vi "Analog Trigger Detect.vi"(8 "acq.Trigger Invert":bool, 9 "acq.Trigger High":i16, 10 "acq.Trigger Low":i16, 11 "Input Data":i16) -> (2 "Analog Trigger Detect":bool, 3 "Analog Arm Trig":bool)   [LabVIEW 2012]
uses:
  <instrlib>/FlexRIO/Libraries/Helper VIs/NI FlexRIO Helper VIs.lvlib
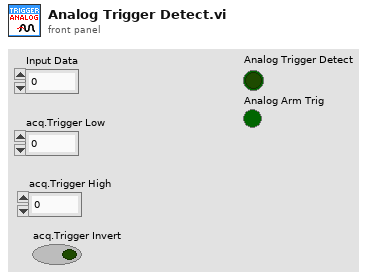
[diagram p1: front panel]
types:
  T1 = cluster{"acq.Trigger Low":i16, "acq.Trigger Invert":bool, "acq.Trigger High":i16}
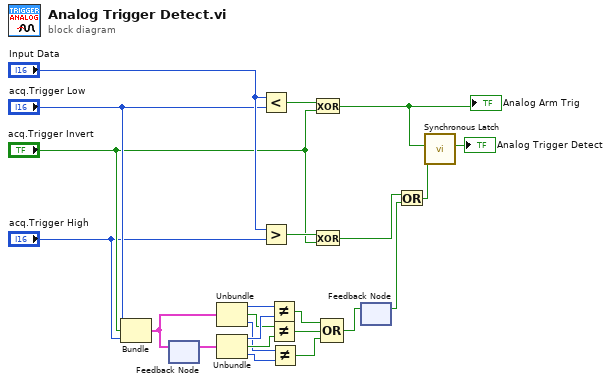
[diagram p0: block diagram]
diagram:
  n1 = Bundle("acq.Trigger Low"="acq.Trigger Low", "acq.Trigger Invert"="acq.Trigger Invert", "acq.Trigger High"="acq.Trigger High") -> (w5:T1)  [unwired: 1 in]
  n2 = feedback #1() -> (w15:T1)  [unwired: 1 in]
  n3 = feedback-in #1(w5) -> ()
  n4 = Unbundle(w5) -> ("acq.Trigger Low"=w13:i16, "acq.Trigger Invert"=w12:bool, "acq.Trigger High"=w7:i16)
  n5 = Unbundle(w15) -> ("acq.Trigger Low"=w14:i16, "acq.Trigger Invert"=w11:bool, "acq.Trigger High"=w6:i16)
  n6 = Less?(x="Input Data", y="acq.Trigger Low") -> (x < y?=w21:bool)
  n7 = Greater?(x="Input Data", y="acq.Trigger High") -> (0:w23:bool)
  n8 = Not Equal?(x=w13, y=w14) -> (x != y?=w9:bool)
  n9 = Not Equal?(x=w12, y=w11) -> (x != y?=w10:bool)
  n10 = Not Equal?(x=w7, y=w6) -> (x != y?=w8:bool)
  n11 = Exclusive Or(1:"acq.Trigger Invert", 2:w21) -> (0:w3:bool)
  "Analog Arm Trig" <- w3
  n12 = Exclusive Or(1:"acq.Trigger Invert", 2:w23) -> (0:w2:bool)
  n13 = Compound Arithmetic op=OR(w9, w10, w8) -> (w4:bool)
  n14 = feedback #2() -> (w16:bool)  [unwired: 1 in]
  n15 = feedback-in #2(w4) -> ()
  n16 = Or(x=w2, y=w16) -> (x .or. y?=w17:bool)
  n17 = call <instrlib>:"Synchronous Latch.vi"("clear"=w17, "set"=w3) -> ("out"=→"Analog Trigger Detect":bool)  [unwired: 9 in]
